vi "DutyCycleOut SetControl.vi"(0 "DeviceReference":T1, 1 "StopSendingOtherRequests":bool=TRUE, 2 "Output":dbl, 3 "EnableFOC":bool=TRUE, 4 "OverrideBrakeDurNeutral":bool, 5 "LimitForwardMotion":bool, 6 "LimitReverseMotion":bool, 7 "error in":errorcluster, 18 "Update Frequency (Hz)":dbl=100.0) -> (20 "DeviceReference Out":T1, 27 "error out":errorcluster)   [LabVIEW 2023]
doc: "Request a specified motor duty cycle.\nThis control mode will output a proportion of the supplied voltage which is supplied by the user."
uses:
  Users/Cory/Documents/PhoenixPro-LabVIEW-Generation/controls/DeviceReference.ctl
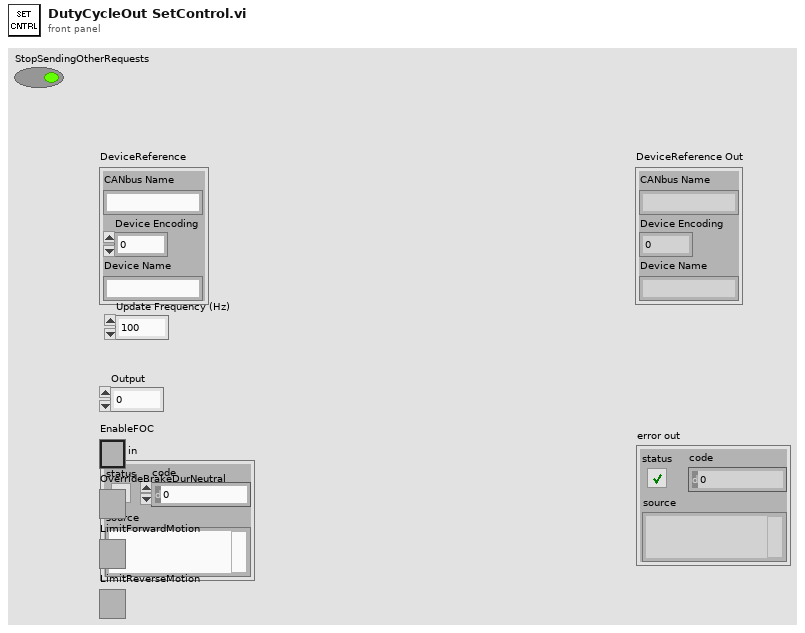
[diagram p1: front panel]
types:
  T1 = typedef "DeviceReference.ctl" = cluster{"CANbus Name":string, "Device Encoding":u32, "Device Name":string}
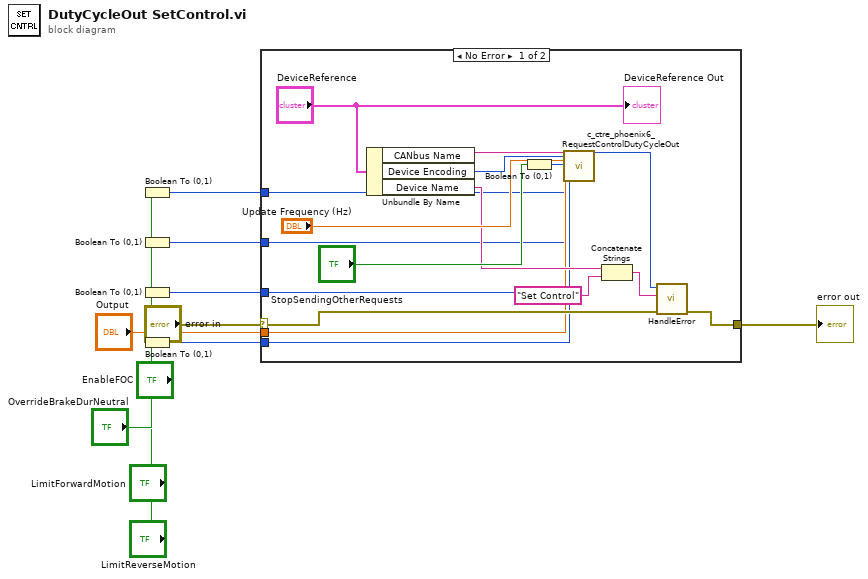
[diagram p0: block diagram]
diagram:
  n1 = Boolean To (0,1)(Boolean="EnableFOC") -> (0, 1=w7:i16)
  n2 = Boolean To (0,1)(Boolean="OverrideBrakeDurNeutral") -> (0, 1=w5:i16)
  n3 = Boolean To (0,1)(Boolean="LimitForwardMotion") -> (0, 1=w3:i16)
  n4 = Boolean To (0,1)(Boolean="LimitReverseMotion") -> (0, 1=w1:i16)
  n5 = case shown="No Error" "error in" {
    selector: "error in" -> [w21 w29]
    tunnel: [w20 w29] -> w10
    tunnel: "Output" -> [w16 _]
    tunnel: w7 -> [w15 _]
    tunnel: w5 -> [w14 _]
    tunnel: w3 -> [w13 _]
    tunnel: w1 -> [w12 _]
    frame No Error {
      n6 = Unbundle By Name("DeviceReference") -> ("CANbus Name"=w27:string, "Device Encoding"=w26:u32, "Device Name"=w19:string)
      n7 = Boolean To (0,1)(Boolean="StopSendingOtherRequests") -> (0, 1=w23:i16)
      n8 = call <vilib>:"c_ctre_phoenix6_RequestControlDutyCycleOut.vi"("String 2"=w27, "Numeric 2"=w26, "Numeric 3"="Update Frequency (Hz)", "Numeric 4"=w23, "Numeric 5"=w16, "Numeric 6"=w15, "Numeric 7"=w14, "Numeric 8"=w13, "Numeric 9"=w12) -> ("Numeric"=w22:i32)  [unwired: 17 in, 1 out]
      n9 = Concatenate Strings(w19, "Set Control" ("origin")) -> (w17:string)
      n10 = call "HandleError.vi"("error in"=w21, "origin"=w17, "Status"=w22) -> ("error out"=w20:errorcluster)  [unwired: 8 in]
      "DeviceReference Out" <- "DeviceReference"
    }
    frame Error {
    }
  }
  "error out" <- w10
